vi "Dialog.vi"() -> (2 "Connection Info out":T1={"host IP"="", "port"=22, "username"="", "password"="", "Connection Name"=""})   [LabVIEW 2017]
uses:
  Libraries/SSH/Connection Info.ctl
  Libraries/SSH/SSH.lvlib
panel:
  in  "OK":bool
  in  "Connection Info":T1={"host IP"="", "port"=22, "username"="", "password"="", "Connection Name"=""}
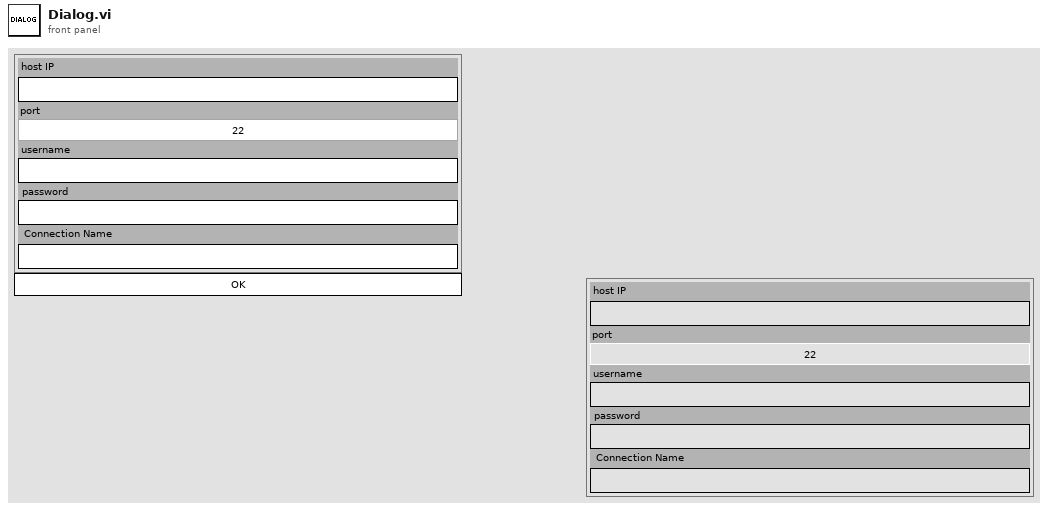
[diagram p1: front panel]
types:
  T1 = typedef "SSH.lvlib/Connection Info.ctl" = cluster{"host IP":string, "port":i32, "username":string, "password":string, "Connection Name":string}
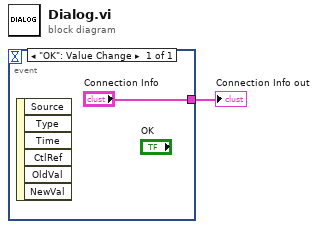
[diagram p0: block diagram]
diagram:
  n1 = event shown="[0] \"OK\": Value Change" {
    selector: _ -> [_]
    dyn-events: _ -> [_]
    timeout: _ -> [_]
    tunnel: ["Connection Info"] -> w1
    event "OK": Value Change {
      n2 = event-data() -> ()  [unwired: 1 in, 6 out]
    }
  }
  "Connection Info out" <- w1
